vi "test_cs.vi"() -> ()   [LabVIEW 2013]
uses:
  lightfield-automation-labview/VIs/ClientServerMode/CS_LFAClassGlobal.vi
  lightfield-automation-labview/LightField Automation.lvclass
panel:
  in  "Delete File?":bool
  in  "Acquire LightField":bool
  out "Acquire LightFiled ROI 1, Frame 1, Row 1":dbl[](graph)
  out "Acquire ROI 1, Frame 1, Row 1":dbl[](graph)
  in  "Acquire":bool
  out "Acquire LightField ROI 1, Frame 1":dbl[][](graph)
  out "Acquire ROI 1, Frame 1":dbl[][](graph)
  in  "?":bool
  out "Exposures Per Frame":i32
  in  "Exposures Per Frame":i32=1
  out "Number of Frames":i32
  in  "Number of Frames":i32=1
  out "Exposure Time (s)":dbl
  in  "Exposure Time (s)":dbl=0.1
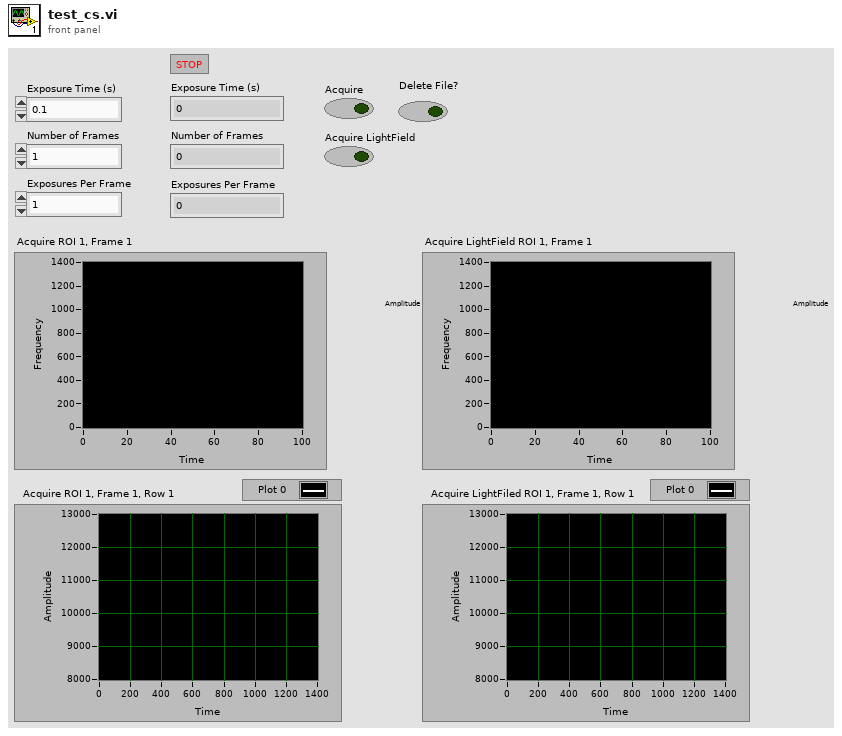
[diagram p1: front panel]
types:
  T1 = cluster{"Image":dbl[][][], "Frame Size":cluster{"F":i32, "Y":i32, "X":i32}}[]
  T2 = cluster{"Image":dbl[][][], "Frame Size":cluster{"F":i32, "Y":i32, "X":i32}}
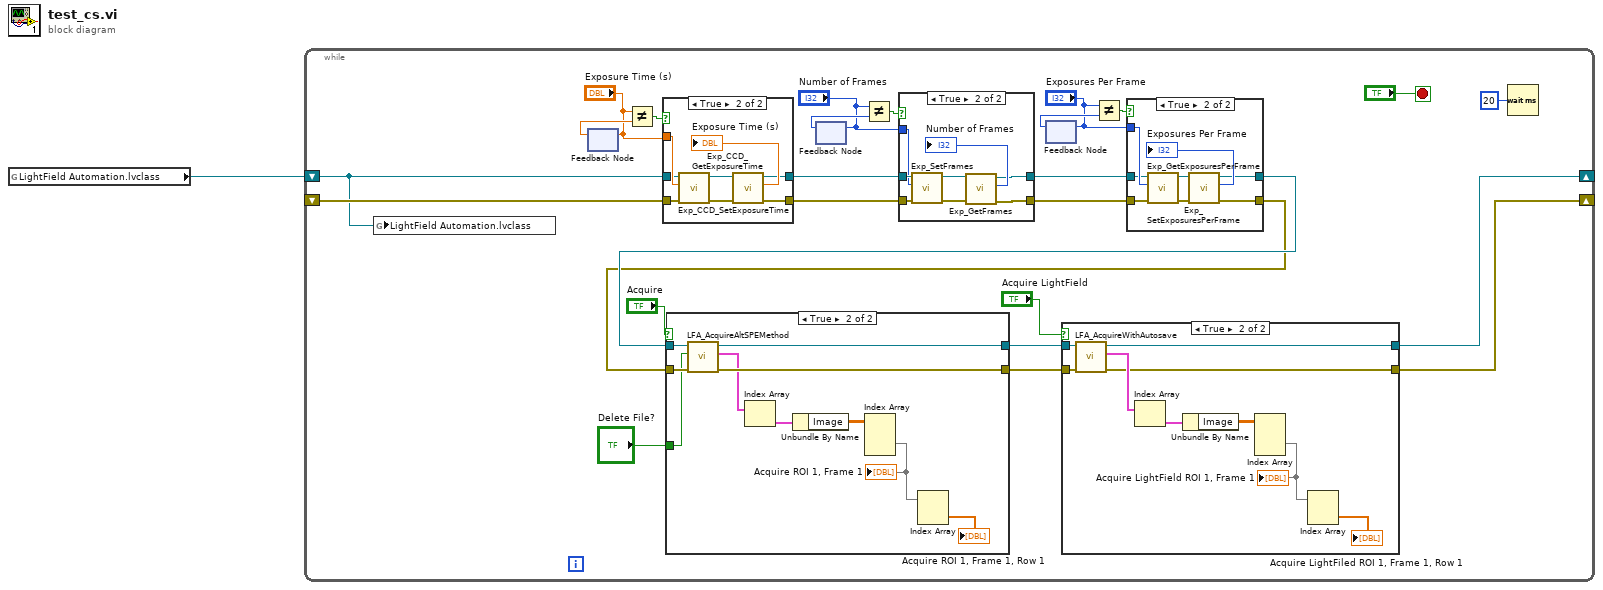
[diagram p0: block diagram]
diagram:
  n1 = global read "CS_LFAClassGlobal.vi" "LightField Automation.lvclass"() -> (w1:refnum<class "LightField Automation.lvclass">)
  n2 = while {
    shift-right: [w7] -> _
    shift-left: w1 -> [w2]
    shift-right: [w6] -> _
    shift-left: _ -> [w3]
    stop <- "?" stop-if-true
    n3 = global write "CS_LFAClassGlobal.vi" "LightField Automation.lvclass"(w2) -> ()
    n4 = feedback-in #1("Exposure Time (s)") -> ()
    n5 = feedback #1() -> (w24:dbl)  [unwired: 1 in]
    n6 = Not Equal?(x="Exposure Time (s)", y=w24) -> (x != y?=w25:bool)
    n7 = case shown="True" w25 {
      tunnel: "Exposure Time (s)" -> [_ w77]
      tunnel: w2 -> [w71 w76]
      tunnel: w3 -> [w72 w75]
      tunnel: [w71 w74] -> w22
      tunnel: [w72 w73] -> w21
      frame False {
      }
      frame True {
        n8 = call "Exp_CCD_SetExposureTime.vi"("error in (no error)"=w75, "Exposure Time (s)"=w77, "LightField Automation in"=w76) -> ("error out"=w78:errorcluster, "LightField Automation out"=w79:refnum<class "LightField Automation.lvclass">)  [unwired: 7 in]
        n9 = call "Exp_CCD_GetExposureTime.vi"("error in (no error)"=w78, "LightField Automation in"=w79) -> ("error out"=w73:errorcluster, "Exposure Time (s)"=→"Exposure Time (s)":dbl, "LightField Automation out"=w74:refnum<class "LightField Automation.lvclass">)  [unwired: 7 in]
      }
    }
    n10 = feedback #2() -> (w20:i32)  [unwired: 1 in]
    n11 = feedback-in #2("Number of Frames") -> ()
    n12 = Not Equal?(x="Number of Frames", y=w20) -> (x != y?=w19:bool)
    n13 = case shown="True" w19 {
      tunnel: w22 -> [w62 w67]
      tunnel: w21 -> [w61 w66]
      tunnel: "Number of Frames" -> [_ w65]
      tunnel: [w62 w64] -> w14
      tunnel: [w61 w63] -> w13
      frame False {
      }
      frame True {
        n14 = call "Exp_SetFrames.vi"("error in (no error)"=w66, "Number of Frames"=w65, "LightField Automation in"=w67) -> ("error out"=w69:errorcluster, "LightField Automation out"=w70:refnum<class "LightField Automation.lvclass">)  [unwired: 7 in]
        n15 = call "Exp_GetFrames.vi"("error in (no error)"=w69, "LightField Automation in"=w70) -> ("error out"=w63:errorcluster, "Frames"=→"Number of Frames":i32, "LightField Automation out"=w64:refnum<class "LightField Automation.lvclass">)  [unwired: 7 in]
      }
    }
    n16 = feedback #3() -> (w17:i32)  [unwired: 1 in]
    n17 = feedback-in #3("Exposures Per Frame") -> ()
    n18 = Not Equal?(x="Exposures Per Frame", y=w17) -> (x != y?=w16:bool)
    n19 = case shown="True" w16 {
      tunnel: "Exposures Per Frame" -> [_ w57]
      tunnel: w14 -> [w52 w56]
      tunnel: w13 -> [w51 w55]
      tunnel: [w51 w54] -> w10
      tunnel: [w52 w53] -> w12
      frame False {
      }
      frame True {
        n20 = call "Exp_SetExposuresPerFrame.vi"("error in (no error)"=w55, "Exposures Per Frame"=w57, "LightField Automation in"=w56) -> ("error out"=w60:errorcluster, "LightField Automation out"=w59:refnum<class "LightField Automation.lvclass">)  [unwired: 7 in]
        n21 = call "Exp_GetExposuresPerFrame.vi"("error in (no error)"=w60, "LightField Automation in"=w59) -> ("error out"=w54:errorcluster, "Exposures Per Frame"=→"Exposures Per Frame":i32, "LightField Automation out"=w53:refnum<class "LightField Automation.lvclass">)  [unwired: 7 in]
      }
    }
    n22 = case shown="True" "Acquire" {
      tunnel: w12 -> [w40 w46]
      tunnel: w10 -> [w39 w45]
      tunnel: [w40 w43] -> w9
      tunnel: [w39 w42] -> w8
      tunnel: "Delete File?" -> [_ w44]
      frame False {
      }
      frame True {
        n23 = call "LFA_AcquireAltSPEMethod.vi"("error in (no error)"=w45, "Delete File?"=w44, "LightField Automation in"=w46) -> ("error out"=w42:errorcluster, "Data"=w41:T1, "LightField Automation out"=w43:refnum<class "LightField Automation.lvclass">)  [unwired: 6 in]
        n24 = Index Array(array=w41) -> (element=w50:T2)  [unwired: 1 in]
        n25 = Unbundle By Name(w50) -> ("Image"=w49:dbl[][][])
        n26 = Index Array(array=w49) -> (element=w48:dbl[][])  [unwired: 3 in]
        "Acquire ROI 1, Frame 1" <- w48
        n27 = Index Array(array=w48) -> (element=→"Acquire ROI 1, Frame 1, Row 1":dbl[])  [unwired: 2 in]
      }
    }
    n28 = case shown="True" "Acquire LightField" {
      tunnel: w9 -> [w29 w33]
      tunnel: w8 -> [w28 w34]
      tunnel: [w29 w32] -> w7
      tunnel: [w28 w30] -> w6
      frame False {
      }
      frame True {
        n29 = call "LFA_AcquireWithAutosave.vi"("error in (no error)"=w34, "LightField Automation in"=w33) -> ("error out"=w30:errorcluster, "Data"=w31:T1, "LightField Automation out"=w32:refnum<class "LightField Automation.lvclass">)  [unwired: 7 in]
        n30 = Index Array(array=w31) -> (element=w38:T2)  [unwired: 1 in]
        n31 = Unbundle By Name(w38) -> ("Image"=w37:dbl[][][])
        n32 = Index Array(array=w37) -> (element=w35:dbl[][])  [unwired: 3 in]
        "Acquire LightField ROI 1, Frame 1" <- w35
        n33 = Index Array(array=w35) -> (element=→"Acquire LightFiled ROI 1, Frame 1, Row 1":dbl[])  [unwired: 2 in]
      }
    }
    n34 = Wait (ms)(milliseconds to wait=u32 20) -> ()  [unwired: 1 out]
  }
